vi "Modify.vi"(7 "Action (noop)":enum8{"noop", "get", "set", "pop"}(ring), 8 "error in (no error)":errorcluster, 10 "skvc input":string[](array[string]), 11 "skvc in":string[][](array[string])) -> (0 "error out":errorcluster, 1 "Found?":bool, 2 "skvc output":string[](array[string]), 3 "skvc out":string[][](array[string]), 4 "Modified?":bool)   [LabVIEW 2018, in "Config.lvlib"]
uses:
  Config.lvlib
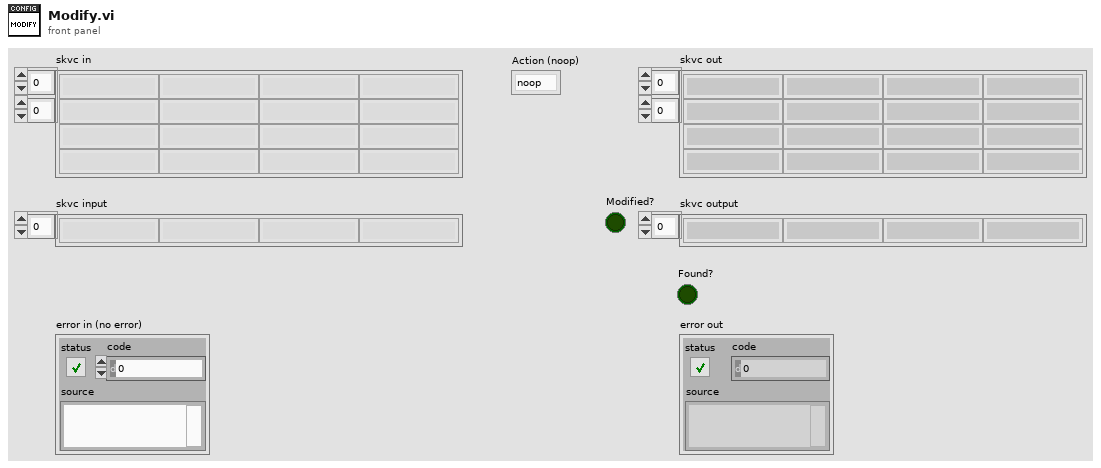
[diagram p1: front panel]
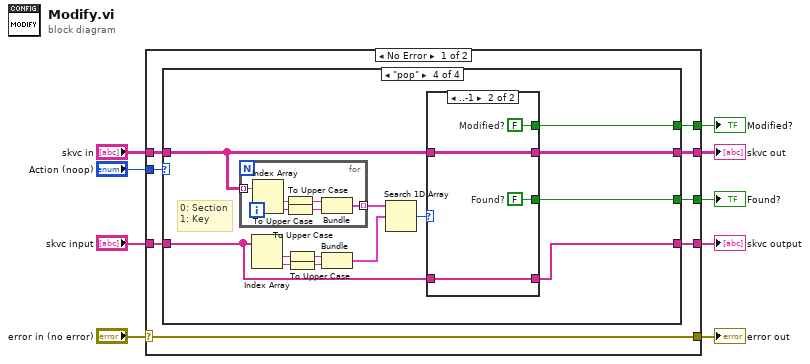
[diagram p0: block diagram]
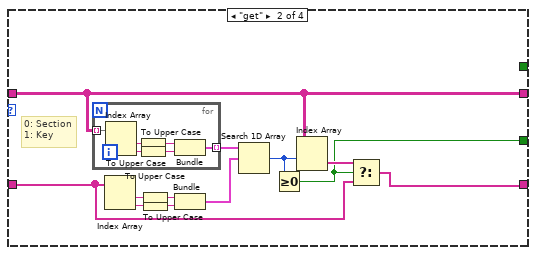
[diagram p3: hidden frame]
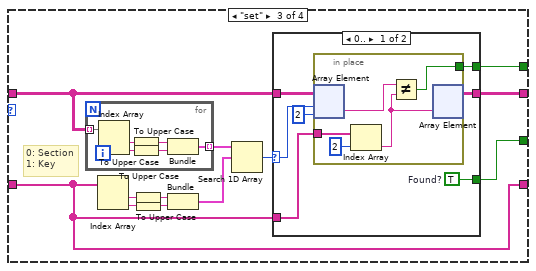
[diagram p4: hidden frame]
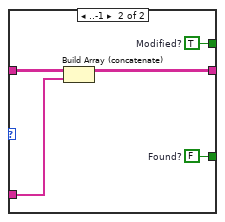
[diagram p5: hidden frame]
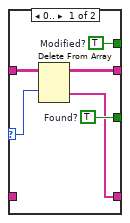
[diagram p6: hidden frame]
diagram:
  n1 = case shown="No Error" "error in (no error)" {
    selector: "error in (no error)" -> [w11 w104]
    tunnel: [w17 _] -> w9
    tunnel: "Action (noop)" -> [w16 _]
    tunnel: "skvc input" -> [w15 w102]
    tunnel: [w14 w102] -> w6
    tunnel: "skvc in" -> [w13 w103]
    tunnel: [w12 w103] -> w4
    tunnel: [w11 w104] -> w3
    tunnel: [w10 _] -> w1
    frame No Error {
      n2 = case shown="\"pop\"" w16 {
        tunnel: w13 -> [w18 w23 w42 w78]
        tunnel: [_ w20 w39 w75] -> w17
        tunnel: w15 -> [w19 w22 w41 w73]
        tunnel: [w19 w21 w41 w74] -> w14
        tunnel: [w18 w23 w40 w77] -> w12
        tunnel: [_ _ w38 w76] -> w10
        frame "noop" {
        }
        frame "get" {
          # "0: Section\n1: Key"
          n3 = for {
            tunnel: w23 -> [w37] mode=indexing
            tunnel: [w34] -> w31 mode=indexing
            n4 = Index Array(array=w37) -> (element #1=w36:string, element #2=w35:string)  [unwired: 2 in]
            n5 = To Upper Case(1:w36) -> (0:w32:string)
            n6 = To Upper Case(1:w35) -> (0:w33:string)
            n7 = Bundle(w32, w33) -> (w34:cluster{string, string})  [unwired: 1 in]
          }
          n8 = Index Array(array=w22) -> (element #1=w25:string, element #2=w24:string)  [unwired: 2 in]
          n9 = To Upper Case(1:w25) -> (0:w30:string)
          n10 = To Upper Case(1:w24) -> (0:w29:string)
          n11 = Bundle(w30, w29) -> (w28:cluster{string, string})  [unwired: 1 in]
          n12 = Search 1D Array(1D array=w31, element=w28) -> (index of element=w27:i32)  [unwired: 1 in]
          n13 = Greater Or Equal To 0?(x=w27) -> (x >= 0?=w20:bool)
          n14 = Index Array(array=w23, index (row)=w27) -> (element=w26:string[])  [unwired: 1 in]
          n15 = Select(t=w26, s=w20, f=w22) -> (s? t:f=w21:string[])
        }
        frame "set" {
          # "0: Section\n1: Key"
          n16 = for {
            tunnel: w42 -> [w72] mode=indexing
            tunnel: [w69] -> w49 mode=indexing
            n17 = Index Array(array=w72) -> (element #1=w71:string, element #2=w70:string)  [unwired: 2 in]
            n18 = To Upper Case(1:w71) -> (0:w67:string)
            n19 = To Upper Case(1:w70) -> (0:w68:string)
            n20 = Bundle(w67, w68) -> (w69:cluster{string, string})  [unwired: 1 in]
          }
          n21 = Index Array(array=w41) -> (element #1=w45:string, element #2=w44:string)  [unwired: 2 in]
          n22 = To Upper Case(1:w45) -> (0:w48:string)
          n23 = To Upper Case(1:w44) -> (0:w47:string)
          n24 = Bundle(w48, w47) -> (w46:cluster{string, string})  [unwired: 1 in]
          n25 = Search 1D Array(1D array=w49, element=w46) -> (index of element=w43:i32)  [unwired: 1 in]
          n26 = case shown="0.." w43 {
            selector: w43 -> [w53 _]
            tunnel: w42 -> [w56 w66]
            tunnel: [w54 w65] -> w40
            tunnel: w41 -> [w52 w64]
            tunnel: [w51 w63] -> w38
            tunnel: [w50 w62] -> w39
            frame 0.. {
              w50 = TRUE  # Found?
              n27 = in-place {
                in-place-border: w52 -> [w61]
                in-place-border: [w57] -> w51
                n28 = in-place-array #1(w56, w53, 2) -> (w59:string)
                n29 = Index Array(array=w61, index=2) -> (element=w58:string)
                n30 = Not Equal?(x=w59, y=w58) -> (x != y?=w57:bool)
                n31 = in-place-array #1(w58) -> (w54:string[][])  [unwired: 2 out]
              }
            }
            frame ..-1 {
              w62 = FALSE  # Found?
              w63 = TRUE  # Modified?
              n32 = Build Array (concatenate)(w66, w64) -> (w65:string[][])
            }
          }
        }
        frame "pop" {
          # "0: Section\n1: Key"
          n33 = for {
            tunnel: w78 -> [w101] mode=indexing
            tunnel: [w98] -> w85 mode=indexing
            n34 = Index Array(array=w101) -> (element #1=w100:string, element #2=w99:string)  [unwired: 2 in]
            n35 = To Upper Case(1:w100) -> (0:w96:string)
            n36 = To Upper Case(1:w99) -> (0:w97:string)
            n37 = Bundle(w96, w97) -> (w98:cluster{string, string})  [unwired: 1 in]
          }
          n38 = Index Array(array=w73) -> (element #1=w81:string, element #2=w80:string)  [unwired: 2 in]
          n39 = To Upper Case(1:w81) -> (0:w84:string)
          n40 = To Upper Case(1:w80) -> (0:w83:string)
          n41 = Bundle(w84, w83) -> (w82:cluster{string, string})  [unwired: 1 in]
          n42 = Search 1D Array(1D array=w85, element=w82) -> (index of element=w79:i32)  [unwired: 1 in]
          n43 = case shown="..-1" w79 {
            selector: w79 -> [w89 _]
            tunnel: w78 -> [w90 w94]
            tunnel: [w87 w92] -> w76
            tunnel: [w91 w95] -> w75
            tunnel: [w88 w94] -> w77
            tunnel: w73 -> [_ w93]
            tunnel: [w86 w93] -> w74
            frame 0.. {
              w87 = TRUE  # Modified?
              w91 = TRUE  # Found?
              n44 = Delete From Array(array=w90, index (row)=w89) -> (deleted portion=w86:string[], array with subset deleted=w88:string[][])  [unwired: 2 in]
            }
            frame ..-1 {
              w92 = FALSE  # Modified?
              w95 = FALSE  # Found?
            }
          }
        }
      }
    }
    frame Error {
    }
  }
  "error out" <- w3
  "skvc out" <- w4
  "skvc output" <- w6
  "Found?" <- w9
  "Modified?" <- w1
